vi "Nidaq_6009_v01.vi"() -> ()   [LabVIEW 2011]
doc: "E-Mail Notification.vi demonstrates a temperature analysis application and how to send a message under certain Limit and Acquistion conditions. This VI asks for recipients for e-mail messages and a valid mail server; reads a simulated temperature; alarms if it is outside a given range;and sends an e-mail referencing condition to listed recipients.\n\nThe Mail Server must be valid for the example to work properly."
panel:
  out "number of samples 4":dbl
  out "mean 4":dbl
  out "min 4":dbl
  out "max 4":dbl
  out "Saida":dbl
  out "number of samples":dbl
  out "mean 3":dbl
  out "min 3":dbl
  out "max 3":dbl
  out "Valvula":dbl
  out "number of samples":dbl
  out "mean 2":dbl
  out "min 2":dbl
  out "max 2":dbl
  out "Entrada":dbl
  out "number of samples":dbl
  out "mean":dbl
  out "min":dbl
  out "max":dbl
  out "Forno":dbl
  out "Time has Elapsed":bool
  out "Temperatura":cluster{dbl, dbl, dbl, dbl}(graph)
  in  "High Limit":dbl(knob)=85.0 scale=70.0..300.0 scale format="%0.0f"
  in  "Low Limit":dbl(knob)=80.07649936341923 scale=0.0..300.0 scale format="%0.0f"
  out "OHL Display":bool
  out "Thermometer":dbl(slide)=79.58984375 scale=70.0..90.0 scale format="%0.2f"
  in  "Acquisition":bool=TRUE
  in  "Update Period":dbl(slide)=1.0 scale=0.0..3.0 scale format="%0.2f"
  out "Temp History":cluster{dbl, dbl, dbl, dbl}(graph)
  # "Temperature History"
  # "System Controls"
  # "Current Temperature"
  # "(deg C)"
  # "(s)"
  # "on\noff"
  # "Temperature Range"
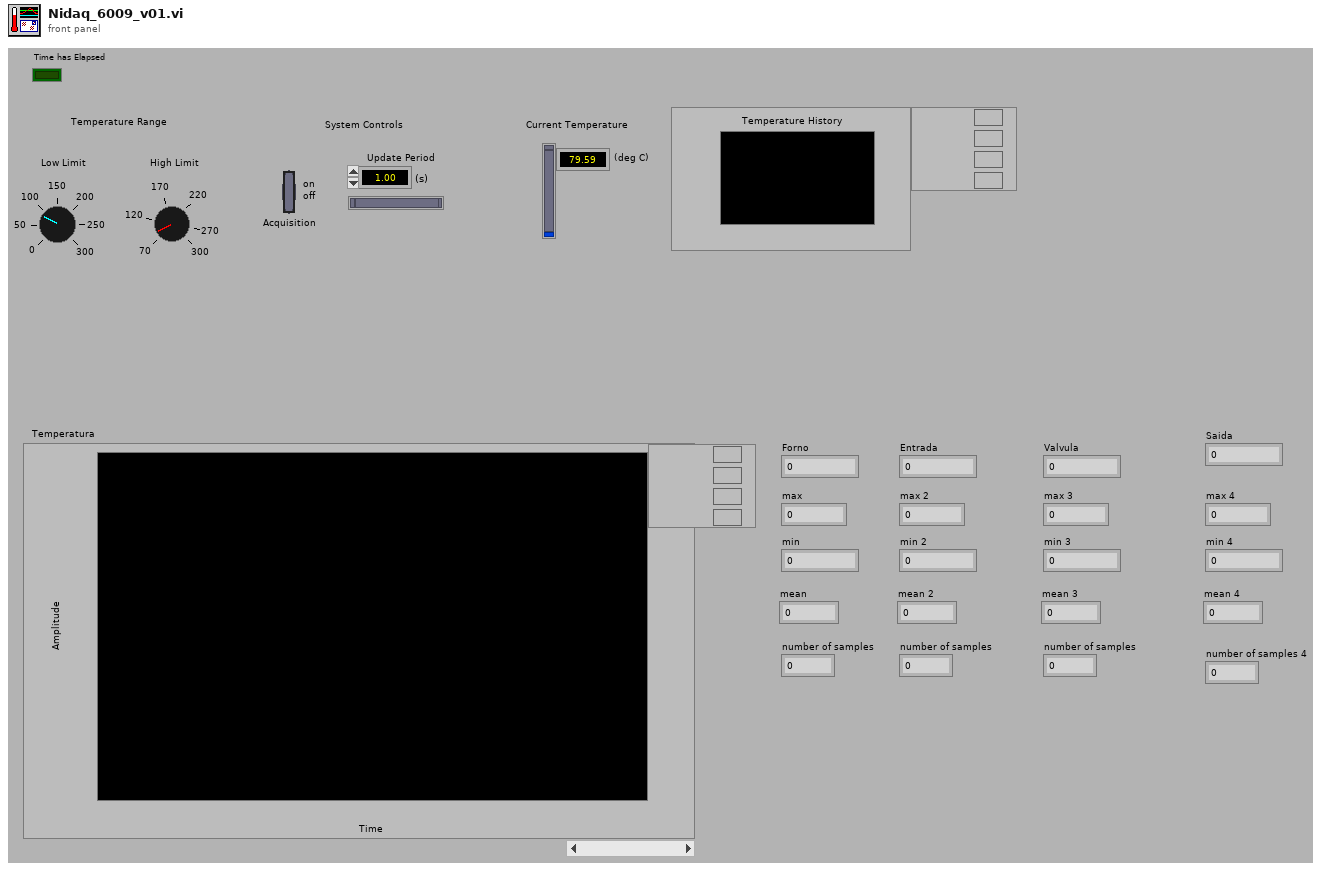
[diagram p1: front panel]
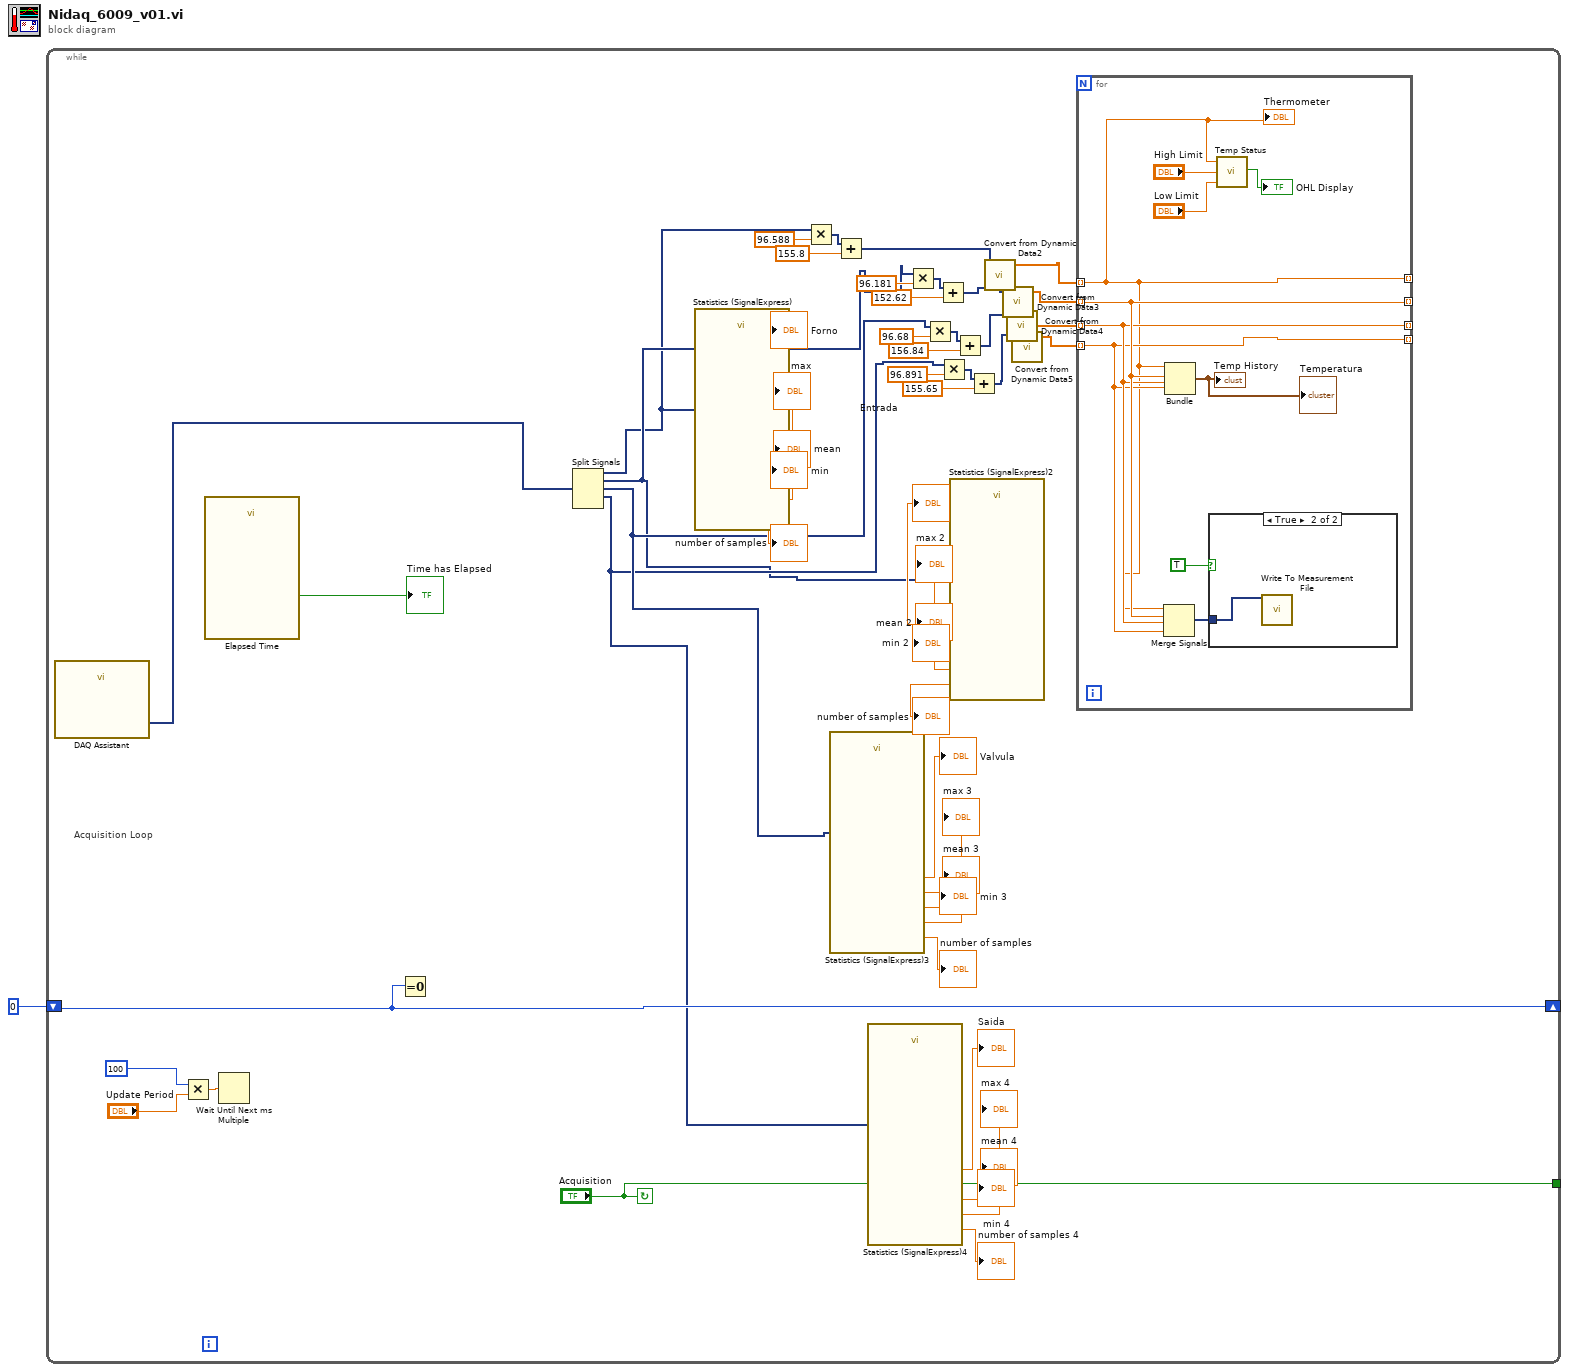
[diagram p0: block diagram]
diagram:
  # "Acquisition Loop"
  n1 = while {
    shift-left: 0 -> [w42]
    shift-right: [w42] -> _
    tunnel: ["Acquisition"] -> _
    stop <- "Acquisition" continue-if-true
    n2 = call "DAQ Assistant"() -> ("data"=w3:dynamicdata)  [unwired: 17 in, 2 out]
    n3 = Multiply(x=100, y="Update Period") -> (x*y=w51:dbl)
    n4 = call "Elapsed Time"() -> ("Time has Elapsed"=→"Time has Elapsed":bool)  [unwired: 12 in, 7 out]
    n5 = Wait Until Next ms Multiple(millisecond multiple=w51) -> ()  [unwired: 1 out]
    n6 = Equal To 0?(x=w42) -> ()  [unwired: 1 out]
    n7 = Split Signals(w3) -> (w2:dynamicdata, w5:dynamicdata, w9:dynamicdata, w7:dynamicdata)  [unwired: 5 in, 1 out]
    n8 = call "Statistics (SignalExpress)"("input signal"=w2) -> ("standard deviation"=→"Forno":dbl, "max"=→"max":dbl, "min"=→"min":dbl, "mean"=→"mean":dbl, "number of samples"=→"number of samples":dbl)  [unwired: 12 in, 2 out]
    n9 = Multiply(x=w2, y=96.588) -> (x*y=w21:dynamicdata)
    n10 = call "Statistics (SignalExpress)3"("input signal"=w9) -> ("standard deviation"=→"Valvula":dbl, "max"=→"max 3":dbl, "min"=→"min 3":dbl, "mean"=→"mean 3":dbl, "number of samples"=→"number of samples":dbl)  [unwired: 12 in, 2 out]
    n11 = Add(x=w21, y=155.8) -> (x+y=w19:dynamicdata)
    n12 = call "Statistics (SignalExpress)4"("input signal"=w7) -> ("standard deviation"=→"Saida":dbl, "max"=→"max 4":dbl, "min"=→"min 4":dbl, "mean"=→"mean 4":dbl, "number of samples"=→"number of samples 4":dbl)  [unwired: 12 in, 2 out]
    n13 = Multiply(x=w5, y=96.181) -> (x*y=w17:dynamicdata)
    n14 = Multiply(x=w9, y=96.68) -> (x*y=w14:dynamicdata)
    n15 = Add(x=w17, y=152.62) -> (x+y=w4:dynamicdata)
    n16 = Multiply(x=w7, y=96.891) -> (x*y=w11:dynamicdata)
    n17 = call "Statistics (SignalExpress)2"("input signal"=w5) -> ("standard deviation"=→"Entrada":dbl, "max"=→"max 2":dbl, "min"=→"min 2":dbl, "mean"=→"mean 2":dbl, "number of samples"=→"number of samples":dbl)  [unwired: 12 in, 2 out]
    n18 = Add(x=w14, y=156.84) -> (x+y=w8:dynamicdata)
    n19 = Add(x=w11, y=155.65) -> (x+y=w6:dynamicdata)
    n20 = call "Convert from Dynamic Data2"("Dynamic Data Type"=w19) -> ("Array"=w26:dbl[])  [unwired: 3 in]
    n21 = call "Convert from Dynamic Data3"("Dynamic Data Type"=w4) -> ("Array"=w25:dbl[])  [unwired: 3 in]
    n22 = call "Convert from Dynamic Data4"("Dynamic Data Type"=w8) -> ("Array"=w24:dbl[])  [unwired: 3 in]
    n23 = call "Convert from Dynamic Data5"("Dynamic Data Type"=w6) -> ("Array"=w23:dbl[])  [unwired: 3 in]
    n24 = for {
      tunnel: [w53] -> _ mode=indexing
      tunnel: w26 -> [w53] mode=indexing
      tunnel: [w59] -> _ mode=indexing
      tunnel: w25 -> [w59] mode=indexing
      tunnel: [w58] -> _ mode=indexing
      tunnel: w24 -> [w58] mode=indexing
      tunnel: [w57] -> _ mode=indexing
      tunnel: w23 -> [w57] mode=indexing
      n25 = Merge Signals(w53, w59, w58, w57) -> (w60:dynamicdata)
      n26 = Bundle(w53, w59, w58, w57) -> (→"Temp History" →"Temperatura":cluster{dbl, dbl, dbl, dbl})  [unwired: 1 out]
      n27 = case shown="True" TRUE {
        tunnel: w60 -> [_ w63]
        frame False {
        }
        frame True {
          n28 = call "Write To Measurement File"("Signals"=w63) -> ()  [unwired: 16 in, 3 out]
        }
      }
      n29 = call "Temp Status.vi"("Low Limit"="Low Limit", "High Limit"="High Limit", "Temperature"=w53) -> ("Over Limit"=→"OHL Display":bool)  [unwired: 2 out]
      "Thermometer" <- w53
    }
  }
